vi "Settings File Path.vi"() -> (3 "settings path":path)   [LabVIEW 2020, in "Manipulator.lvlib"]
uses:
  Manipulator.lvlib
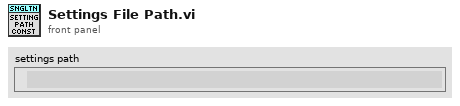
[diagram p1: front panel]
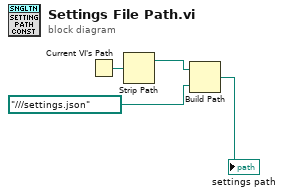
[diagram p0: block diagram]
diagram:
  n1 = Current VI's Path() -> (path=w2:path)
  n2 = Strip Path(path=w2) -> (stripped path=w3:path)  [unwired: 1 out]
  n3 = Build Path(base path=w3, name or relative path=path "../../../settings.json") -> (appended path=→"settings path":path)
